vi "2_图片读取与保存_un.vi"() -> ()   [LabVIEW 2020]
panel:
  in  "停止运行":bool
  out "找到图片":bool
  in  "File Path":path
  out "error out":errorcluster
  out "Image":T1(plugin-control)
  in  "Image Type":T2 items=["Grayscale (U8)", "Grayscale (I16)", "Grayscale (SGL)", "Complex (CSG)", "RGB (U32)", "HSL (U32)", "RGB (U64)", "Grayscale (U16)"]
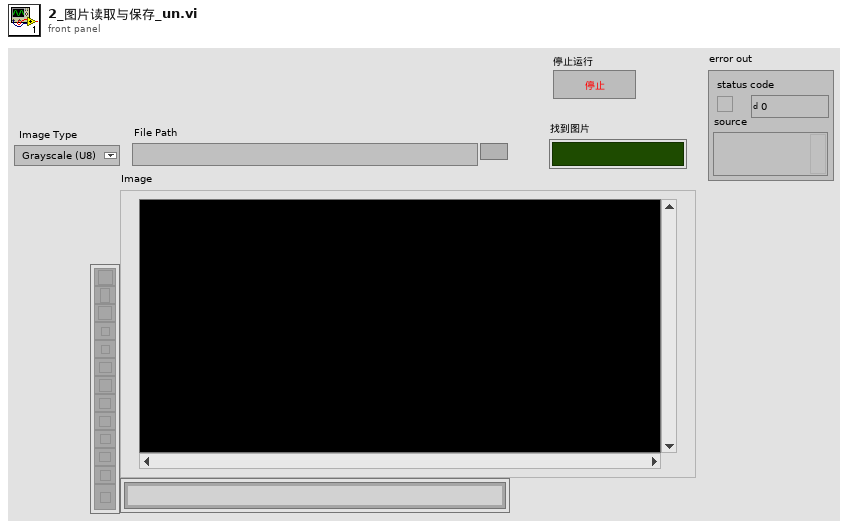
[diagram p1: front panel]
types:
  T1 = typedef "IMAQ Image.ctl" = refnum<image>
  T2 = typedef "Image Type" = u32
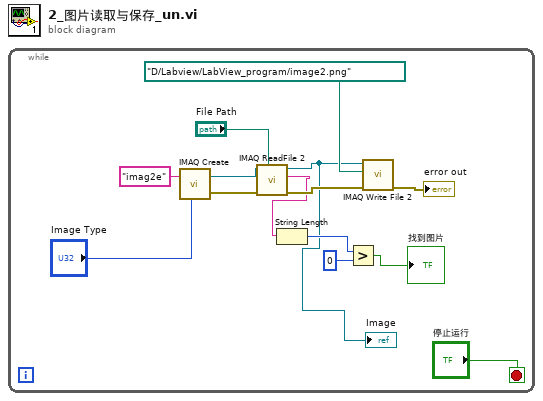
[diagram p0: block diagram]
diagram:
  n1 = while {
    stop <- "停止运行" stop-if-true
    n2 = call "IMAQ Create"("Image Name"="imag2e", "Image Type"="Image Type") -> ("New Image"=w2:T1, "error out"=w12:errorcluster)  [unwired: 3 in]
    n3 = call "IMAQ ReadFile 2"("File Path"="File Path", "error in (no error)"=w12, "Image"=w2) -> ("error out"=w11:errorcluster, "File Type out"=w5:string, "Image Out"=w1:T1)  [unwired: 4 in, 2 out]
    "Image" <- w1
    n4 = String Length(string=w5) -> (length=w7:i32)
    n5 = Greater?(x=w7, y=0) -> (0:→"找到图片":bool)
    n6 = call-poly "IMAQ Write File 2"("error in (no error)"=w11, "File Path"=path "D:/Labview/LabView_program/image2.png", "Image"=w1) -> ("error out"=→"error out":errorcluster)  [unwired: 7 in, 1 out]
  }
